vi "Send Aircraft Heartbeat.vi"(8 "error in (no error)":errorcluster, 11 "Aircraft ID":u8) -> ()   [LabVIEW 2014]
uses:
  Aircraft Information/Sub VI/Get Aircraft RC Override.vi
  Application Support/Stop Button/SubVI/Get Stop Button Status.vi
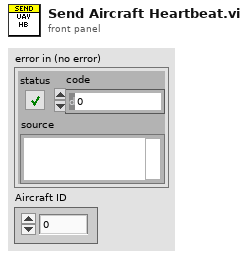
[diagram p1: front panel]
types:
  T1 = typedef "RC Override.ctl" = cluster{"Throttle":u16, "Roll":u16, "Pitch":u16, "Yaw":u16, "Arm":bool, "Disarm":bool, "Aircraft Mode":T2}
  T2 = typedef "Aircraft Mode.ctl" = enum16{"Loiter", "Stabalise", "Failsafe", "Emergency Stop"}
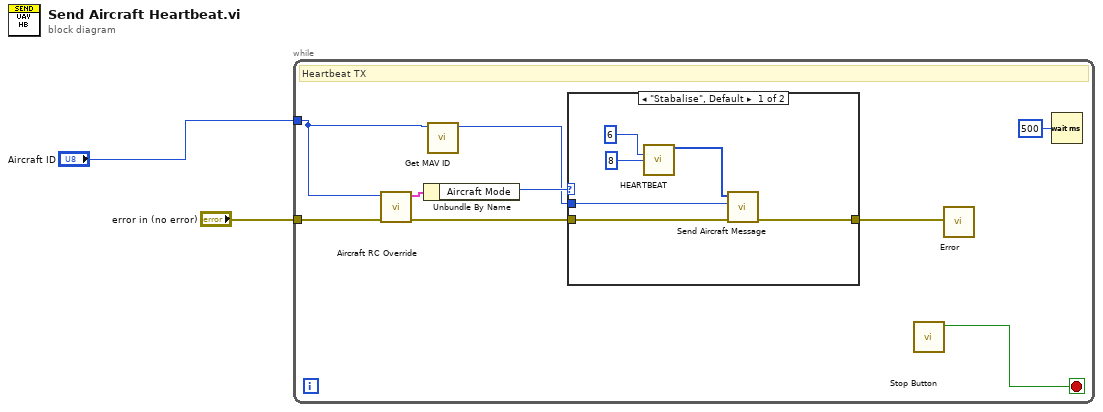
[diagram p0: block diagram]
diagram:
  n1 = while {
    tunnel: "error in (no error)" -> [w8]
    tunnel: "Aircraft ID" -> [w4]
    stop <- w11 stop-if-true
    # "Heartbeat TX"
    n2 = call-poly "Aircraft RC Override.vi"("Error In"=w8, "Aircraft ID"=w4) -> ("Error Out"=w7:errorcluster, "RC Override Values Out"=w6:T1)  [unwired: 8 in]
    n3 = Unbundle By Name(w6) -> ("Aircraft Mode"=w5:T2)
    n4 = call "Get MAV ID.vi"("Aircraft Index"=w4) -> ("Aircraft ID"=w3:u8)  [unwired: 9 in, 1 out]
    n5 = case shown="\"Stabalise\", Default" w5 {
      tunnel: w7 -> [w17 w18]
      tunnel: [w13 w18] -> w9
      tunnel: w3 -> [w12 _]
      frame "Stabalise", Default {
        n6 = call "HEARTBEAT.vi"("type"=u8 6, "autopilot"=u8 8) -> ("MAVLink Message"=w16:u8[])  [unwired: 13 in]
        n7 = call "Send Aircraft Message.vi"("error in (no error)"=w17, "Aircraft ID"=w12, "MAVLink Message"=w16) -> ("error out"=w13:errorcluster)  [unwired: 8 in]
      }
      frame "Failsafe" {
        # "Stop Sending Heartbeat"
      }
    }
    n8 = call-poly "Stop Button.vi"() -> ("Stop ButtonOut"=w11:bool)  [unwired: 10 in, 1 out]
    n9 = call "Error.vi"("Error In"=w9) -> ()  [unwired: 10 in, 1 out]
    n10 = Wait (ms)(milliseconds to wait=u32 500) -> ()  [unwired: 1 out]
  }
